vi "LABVIEW output arduino.vi"() -> ()   [LabVIEW 2023]
uses:
  <vilib>/Instr/_visa.llb/VISA Configure Serial Port (Instr).vi
panel:
  out "Totale hoeveelheid uitgespoten water (mL)":dbl
  out "Watersnelheid (L/min)":dbl
  in  "stop":bool
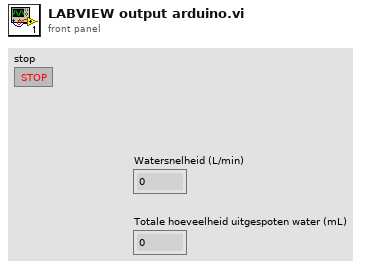
[diagram p1: front panel]
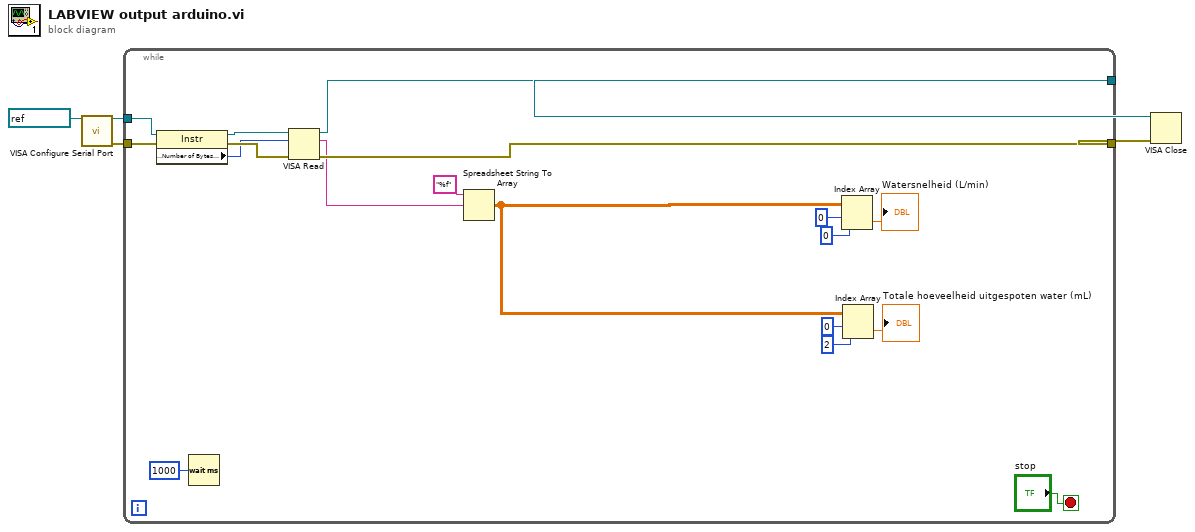
[diagram p0: block diagram]
diagram:
  n1 = call-poly "VISA Configure Serial Port"("VISA resource name"=refnum<visa-resource-name> "COM7") -> ("VISA resource name out"=w4:refnum<visa-resource-name>, "error out"=w1:errorcluster)  [unwired: 13 in]
  n2 = while {
    tunnel: w4 -> [w23]
    tunnel: [w21] -> w3
    tunnel: [w20] -> w2
    tunnel: w1 -> [w18]
    stop <- "stop" stop-if-true
    n3 = property class="Instr"(reference=w23, error in=w18) -> (reference out=w22:refnum<visa-resource-name>, error out=w19:errorcluster, "Serial Settings:Number of Bytes at Serial Port"=w17:u32)
    n4 = Wait (ms)(milliseconds to wait=u32 1000) -> ()  [unwired: 1 out]
    n5 = VISA Read(VISA resource name=w22, byte count=w17, error in (no error)=w19) -> (VISA resource name out=w21:refnum<visa-resource-name>, read buffer=w15:string, error out=w20:errorcluster)  [unwired: 1 out]
    n6 = Spreadsheet String To Array(format string="%f", spreadsheet string=w15) -> (array=w12:dbl[][])  [unwired: 2 in]
    n7 = Index Array(array=w12, index (row)=0, index (col)=0 ("disabled index (col)")) -> (element=→"Watersnelheid (L/min)":dbl)
    n8 = Index Array(array=w12, index (row)=0, index (col)=2 ("disabled index (col)")) -> (element=→"Totale hoeveelheid uitgespoten water (mL)":dbl)
  }
  n9 = VISA Close(VISA resource name=w3, error in (no error)=w2) -> ()  [unwired: 1 out]
